vi "shutDownHW.vi"(8 "error in (no error)":errorcluster, 11 "CompactRIO in":refnum<class "CompactRIO.lvclass">) -> (0 "error out":errorcluster, 3 "CompactRIO out":refnum<class "CompactRIO.lvclass">)   [LabVIEW 2015, in "CompactRIO.lvclass"]
doc: "Performs any operations necessary to shut down the hardware. For a cRIO target it aborts the FPGA VI."
uses:
  CompactRIO.lvclass
  CompactRIO.lvclass/CompactRIO.ctl
  <vilib>/FPGAPlugInAG/cRIO-9074/niLvFpga_Abort_cRIO-9074.vi
  <vilib>/FPGAPlugInAG/cRIO-9074/niLvFpga_Close_cRIO-9074.vi
  <vilib>/rvi/interface/nirviMethod/nirviMethod.xnode
  ComponentTemplateCore/ComponentModel/ComponentModelRT/Typedefs/FPGAVIRefCRIO9074.ctl
  <vilib>/rvi/interface/nirviCloseFPGA/nirviCloseFPGA.xnode
  fpgaVIReference.ctl
  FPGA Bitfiles/cRIOApp_FPGATarget_fpgaMain_F827BADB.lvbitx
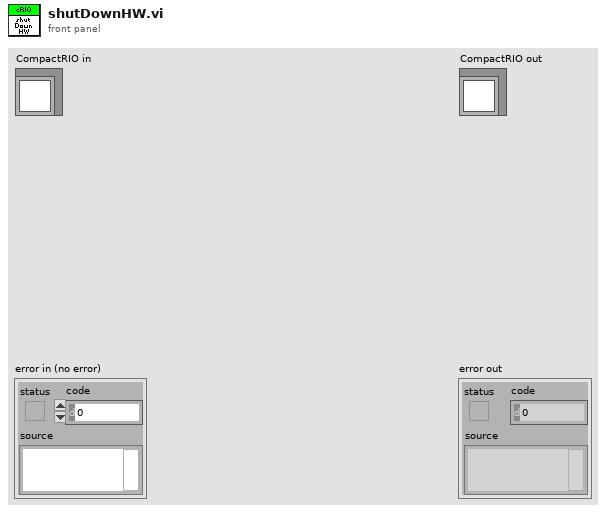
[diagram p1: front panel]
types:
  T1 = typedef "fpgaVIRefCRIO9074.ctl" = refnum<k20>
  T2 = typedef "fpgaVIReference.ctl" = refnum<k20>
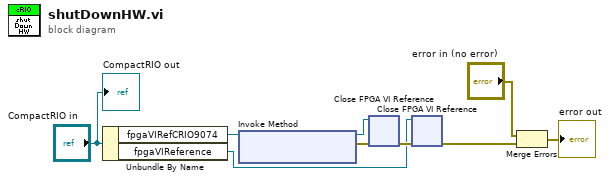
[diagram p0: block diagram]
diagram:
  n1 = Unbundle By Name("CompactRIO in") -> ("fpgaVIRefCRIO9074"=w9:T1, "fpgaVIReference"=w3:T2)
  n2 = xnode "Invoke Method"("FPGA VI Reference In"=w9) -> ("FPGA VI Reference Out"=w5:T1, "error out"=w2:errorcluster)  [unwired: 1 in]
  n3 = xnode "Close FPGA VI Reference"("FPGA VI Reference In"=w5, "error in"=w2) -> ("error out"=w4:errorcluster)
  n4 = xnode "Close FPGA VI Reference"("FPGA VI Reference In"=w3, "error in"=w4) -> ("error out"=w1:errorcluster)
  n5 = Merge Errors("error in (no error)", w1) -> (→"error out":errorcluster)
  "CompactRIO out" <- "CompactRIO in"
